vi "Configure Port Impedance Conversion.vi"(0 "VISA resource name":refnum<visa-resource-name>, 1 "Channel (1)":i32=1, 2 "Fixture Simulator Function State (F: Disable)":bool, 3 "Port 1 (1)":i32=1, 5 "Circuit Mode (0: Normal)":u16(ring) items=["Normal", "Differential", "Common"], 11 "error in (no error)":errorcluster, 12 "Z0 (50.0)":dbl=50.0 format="%.2f") -> (4 "VISA resource name out":refnum<visa-resource-name>, 15 "error out":errorcluster)   [LabVIEW 2011, in "Agilent ENA Series.lvlib"]
doc: "This VI configures port impedance conversion."
uses:
  Agilent ENA Series.lvlib
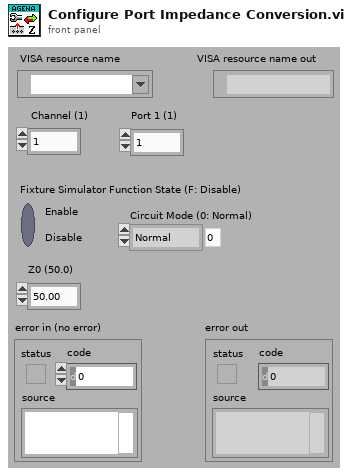
[diagram p1: front panel]
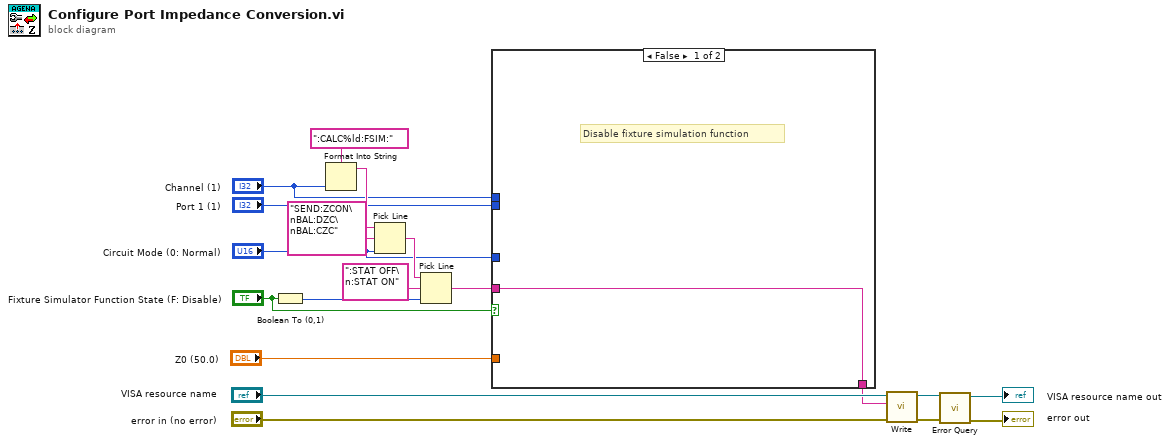
[diagram p0: block diagram]
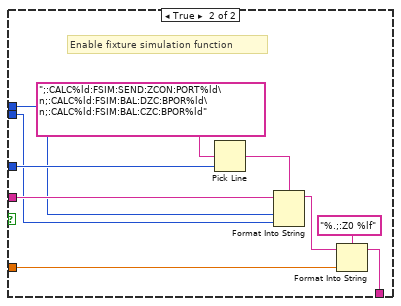
[diagram p2: hidden frame]
diagram:
  n1 = Boolean To (0,1)(Boolean="Fixture Simulator Function State (F: Disable)") -> (0, 1=w13:i16)
  n2 = Format Into String(format string=":CALC%ld:FSIM:", "Channel (1)") -> (resulting string=w15:string)  [unwired: 2 in, 1 out]
  n3 = Pick Line(string ("")=w15, multi-line string="SEND:ZCON\nBAL:DZC\nBAL:CZC", line index="Circuit Mode (0: Normal)") -> (output string=w12:string)
  n4 = Pick Line(string ("")=w12, multi-line string=":STAT OFF\n:STAT ON", line index=w13) -> (output string=w7:string)
  n5 = case shown="False" "Fixture Simulator Function State (F: Disable)" {
    tunnel: "Circuit Mode (0: Normal)" -> [_ w27]
    tunnel: "Channel (1)" -> [_ w26]
    tunnel: "Port 1 (1)" -> [_ w25]
    tunnel: w7 -> [w20 w28]
    tunnel: "Z0 (50.0)" -> [_ w23]
    tunnel: [w20 w21] -> w5
    frame False {
      # "Disable fixture simulation function"
    }
    frame True {
      # "Enable fixture simulation function"
      n6 = Pick Line(multi-line string=";:CALC%ld:FSIM:SEND:ZCON:PORT%ld\n;:CALC%ld:FSIM:BAL:DZC:BPOR%ld\n;:CALC%ld:FSIM:BAL:CZC:BPOR%ld", line index=w27) -> (output string=w29:string)  [unwired: 1 in]
      n7 = Format Into String(format string=w29, initial string=w28, w26, w25) -> (resulting string=w22:string)  [unwired: 1 in, 1 out]
      n8 = Format Into String(format string="%.;:Z0 %lf", initial string=w22, w23) -> (resulting string=w21:string)  [unwired: 1 in, 1 out]
    }
  }
  n9 = call "Write.vi"("error in (no error)"="error in (no error)", "String ()"=w5, "VISA resource name"="VISA resource name") -> ("error out"=w3:errorcluster, "VISA resource name out"=w4:refnum<visa-resource-name>)  [unwired: 6 in, 1 out]
  n10 = call "Error Query.vi"("error in (no error)"=w3, "VISA resource name"=w4) -> ("error out"=→"error out":errorcluster, "VISA resource name out"=→"VISA resource name out":refnum<visa-resource-name>)  [unwired: 6 in, 2 out]
